vi "IdentifyHP5385A.vi"(8 "error in (no error)":errorcluster, 11 "VISA Resource Name":refnum<visa-resource-name>) -> (0 "error out":errorcluster, 2 "Identified":bool, 3 "VISA Resource Name Out":refnum<visa-resource-name>)   [LabVIEW 2015]
uses:
  GPIB/VISA  Send Receive.vi
panel:
  out "data":string
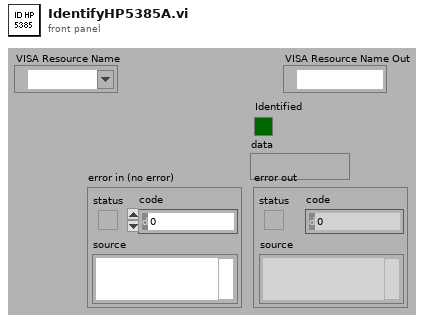
[diagram p1: front panel]
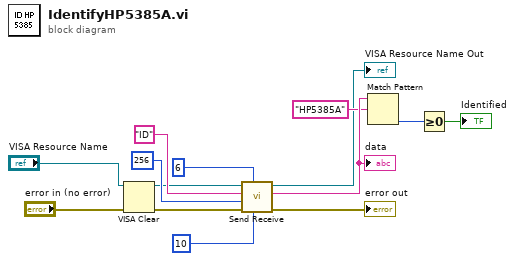
[diagram p0: block diagram]
diagram:
  n1 = VISA Clear(VISA resource name="VISA Resource Name", error in (no error)="error in (no error)") -> (VISA resource name out=w2:refnum<visa-resource-name>, error out=w5:errorcluster)
  n2 = call-poly "Send Receive.vi"("Read terminator"=i16 10, "Delay, ms"=u32 6, "error in (no error)"=w5, "Receive count"=256 ("byte count"), "data string in"="ID", "VISA Resource Name"=w2) -> ("error out"=→"error out":errorcluster, "data string out"=w10:string, "VISA Resource Name Out"=→"VISA Resource Name Out":refnum<visa-resource-name>)  [unwired: 3 in]
  "data" <- w10
  n3 = Match Pattern(string=w10, regular expression="HP5385A") -> (offset past match=w8:i32)  [unwired: 4 out]
  n4 = Greater Or Equal To 0?(x=w8) -> (x >= 0?=→"Identified":bool)
